vi "Handle Response.vi"(7 "Processing In":refnum<class "Processing.lvclass">, 11 "WebSocket Handler in":refnum<class "WebSocket Handler.lvclass">) -> (0 "error out":errorcluster, 5 "Processing":refnum<class "Processing.lvclass">)   [LabVIEW 2020, in "HTTP Server.lvlib" / "WebSocket Handler.lvclass"]
uses:
  WebSocket Handler.lvclass
  WebSocket Handler.lvclass/WebSocket Handler.ctl
  Processing/Processing.lvclass
  WebSocket Client/WebSocket Client.lvclass
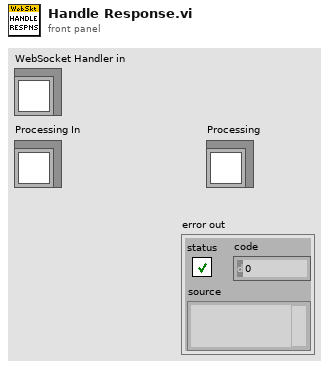
[diagram p1: front panel]
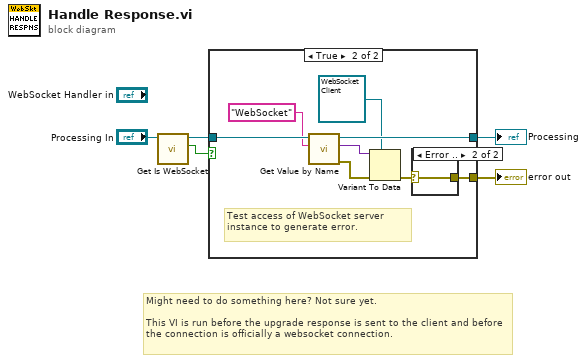
[diagram p0: block diagram]
diagram:
  # "Might need to do something here? Not sure yet.\n\nThis VI is run before the upgrade response is sent to the client and before the connection is officially a websocket connection."
  n1 = call "Get Is WebSocket.vi"("Processing in"="Processing In") -> ("Is WebSocket"=w3:bool, "Processing out"=w4:refnum<class "Processing.lvclass">)  [unwired: 9 in]
  n2 = case shown="True" w3 {
    tunnel: w4 -> [w6 w14]
    tunnel: [w6 w12] -> w2
    tunnel: [_ w11] -> w1
    frame False {
    }
    frame True {
      # "Test access of WebSocket server instance to generate error."
      n3 = call "Get Value by Name.vi"("Name"="WebSocket" ("Name for Type"), "Processing in"=w14) -> ("error out"=w9:errorcluster, "Value"=w10:variant, "Processing out"=w12:refnum<class "Processing.lvclass">)  [unwired: 7 in]
      n4 = Variant To Data(error in=w9, type=refnum<class "WebSocket Client.lvclass"> refnum ("WebSocket"), Variant=w10) -> (error out=w7:errorcluster)  [unwired: 1 out]
      n5 = case shown="Error .." w7 {
        selector: w7 -> [w15 w16]
        tunnel: [w15 w16] -> w11
        frame No Error {
        }
        frame Error {
        }
      }
    }
  }
  "error out" <- w1
  "Processing" <- w2
